vi "Create Container.vi"(8 "Error In":errorcluster, 11 "Abstract Widget Builder in":refnum<class "Abstract Widget Builder.lvclass">) -> (0 "Error Out":errorcluster, 2 "Container":refnum<class "QWidget.lvclass">, 3 "Abstract Widget Builder out":refnum<class "Abstract Widget Builder.lvclass">)   [LabVIEW 2014, in "Abstract Widget Builder.lvclass"]
doc: "Creates a new \"container\" for a Growable Widget and adds a single chart widget to the container.\n\nThis VI must be overridden by descendent classes.\n\n\nCopyright (c) 2019 Sze Howe Koh.\nThis code is licensed under the MIT license."
uses:
  Abstract Widget Builder.lvclass
  <vilib>/addons/LQ/Qt Widgets/QWidget/QWidget.lvclass
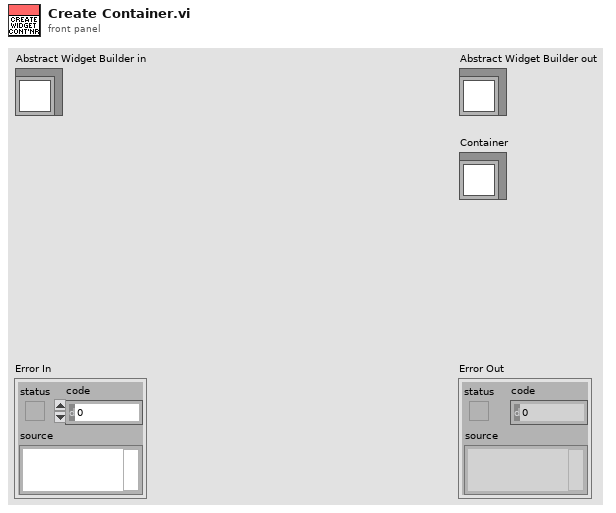
[diagram p1: front panel]
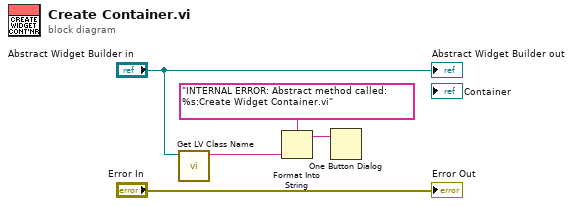
[diagram p0: block diagram]
diagram:
  n1 = call <vilib>:"Get LV Class Name.vi"("object"="Abstract Widget Builder in") -> ("class name"=w2:string)  [unwired: 9 in, 1 out]
  n2 = Format Into String(format string="INTERNAL ERROR: Abstract method called:  %s:Create Widget Container.vi" ("message"), w2) -> (resulting string=w1:string)  [unwired: 2 in, 1 out]
  n3 = One Button Dialog(message=w1) -> ()  [unwired: 1 in, 1 out]
  "Error Out" <- "Error In"
  "Abstract Widget Builder out" <- "Abstract Widget Builder in"
